vi "QPSK Demodulation (SubVI).vi"(11 "Array in":dynamicdata[](array[waveform])) -> (1 "Output bits":dbl[](array[numeric]), 2 "Constellation graph":cluster{"Y":dbl[], "Y":dbl[]}[](graph), 3 "Even bits":dbl[](graph), 4 "size(s)":i32, 5 "Odd bits":dbl[](graph), 6 "output bits graph":dbl[](graph))   [LabVIEW 2026]
uses:
  <vilib>/measure/madcrms.llb/Basic Averaged DC-RMS for N Chan.vi
  <vilib>/measure/NI_MAPro.lvlib
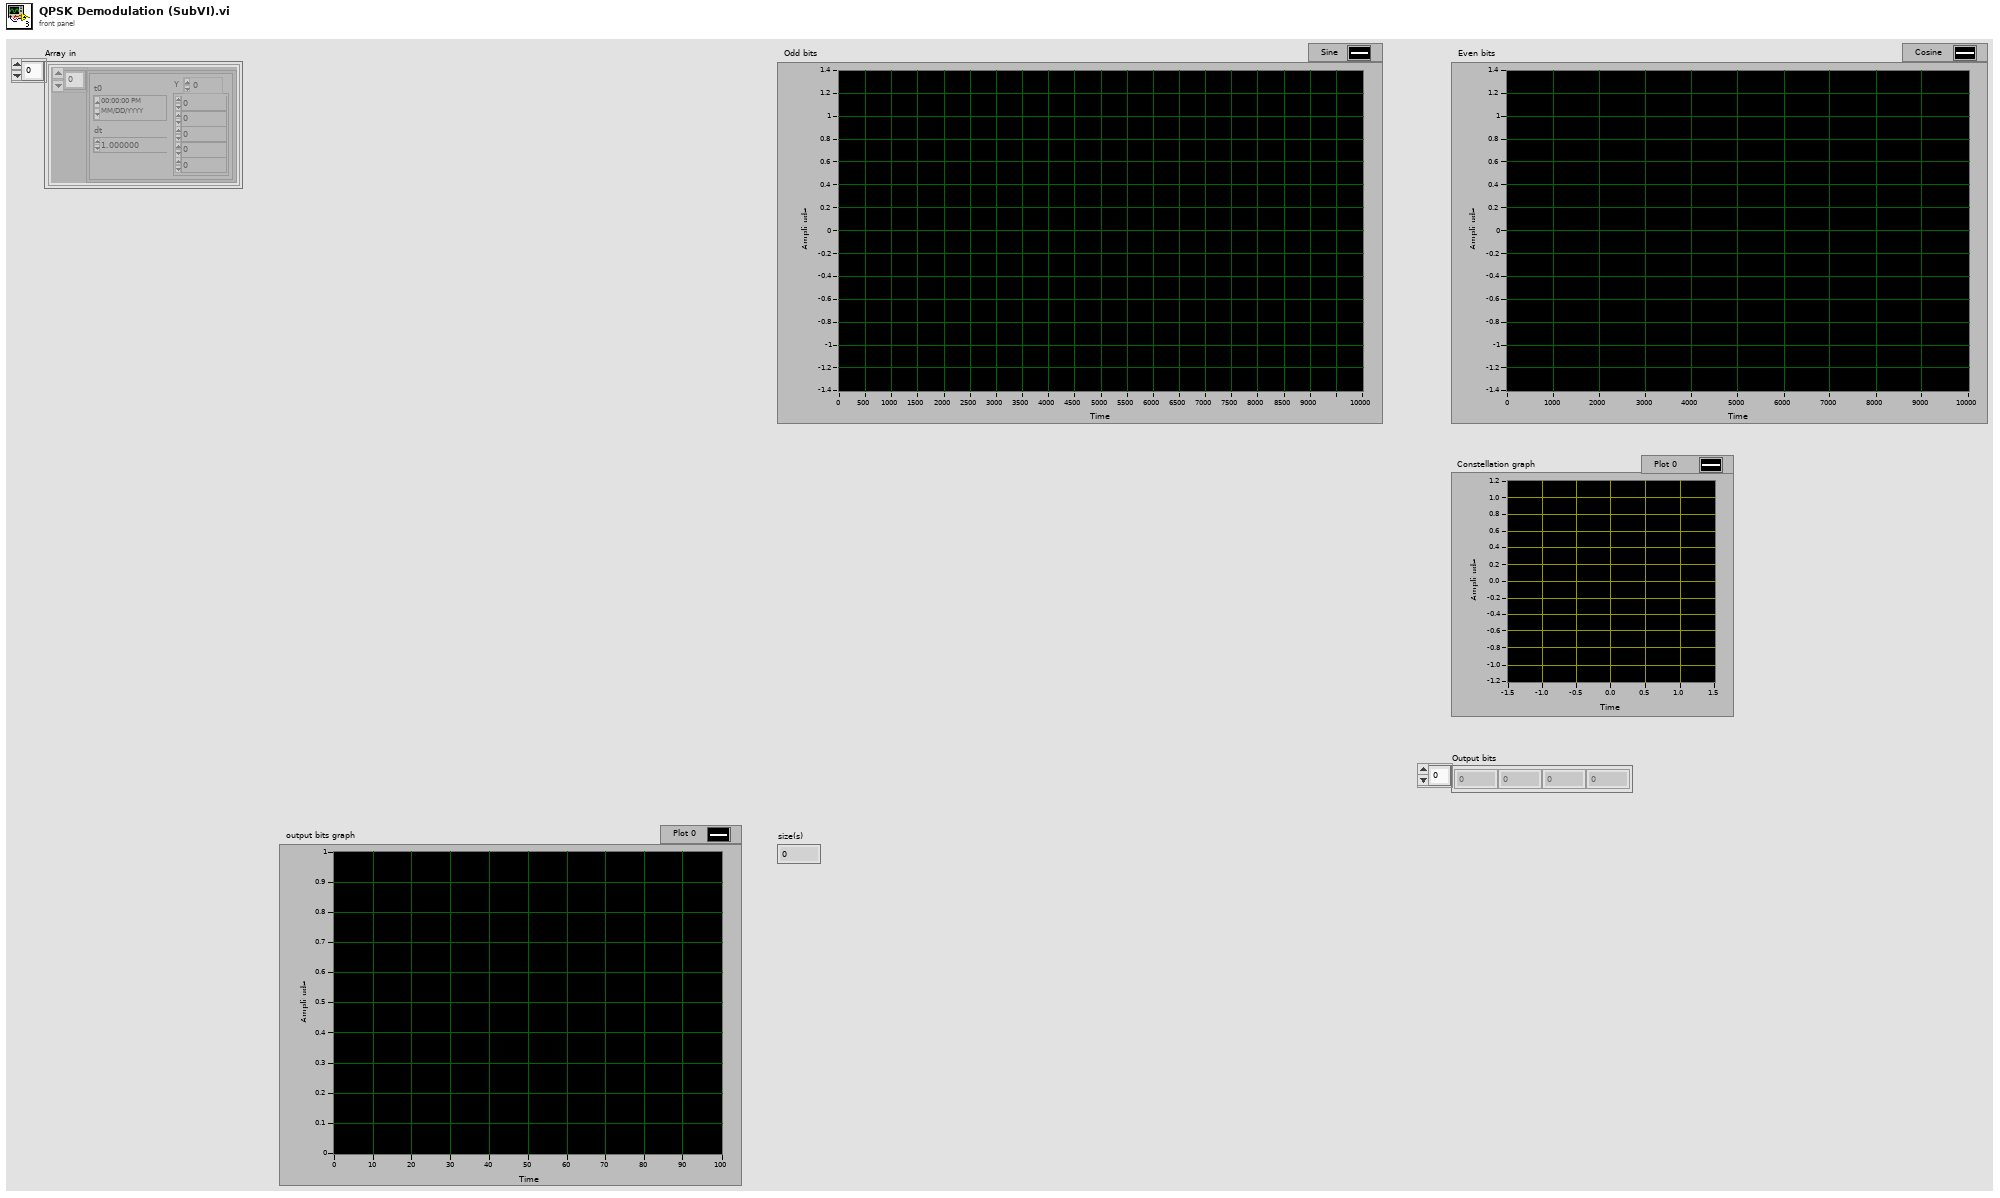
[diagram p1: front panel]
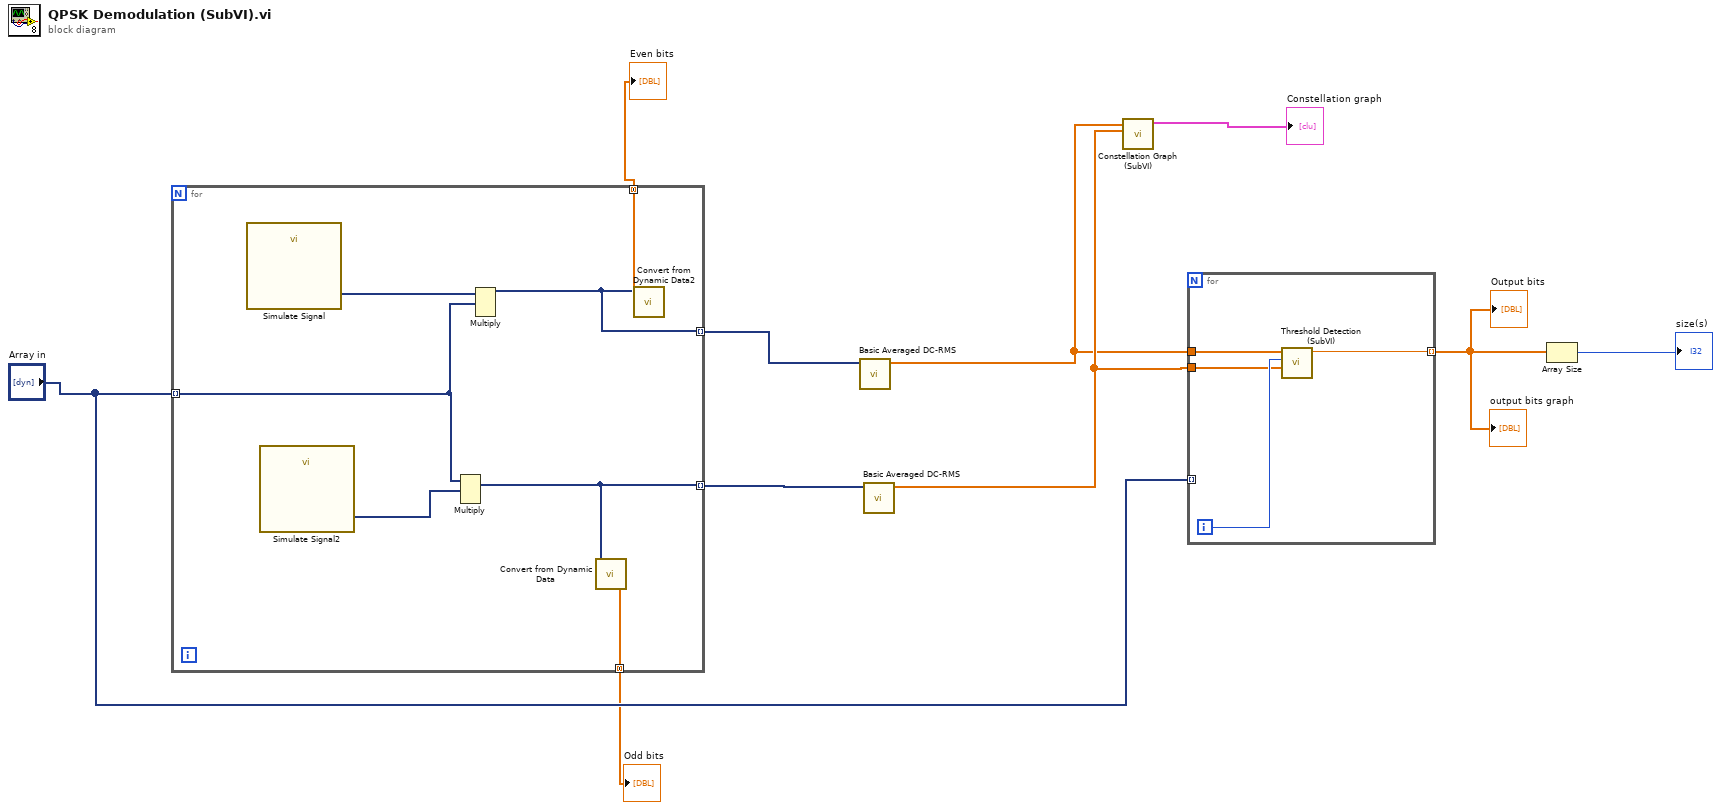
[diagram p0: block diagram]
diagram:
  n1 = for {
    tunnel: "Array in" -> [w15] mode=indexing
    tunnel: [w13] -> w4 mode=concatenating
    tunnel: [w14] -> w3 mode=concatenating
    tunnel: [w12] -> w5 mode=indexing
    tunnel: [w11] -> w6 mode=indexing
    n2 = call "Simulate Signal"() -> ("Cosine"=w17:dynamicdata)  [unwired: 14 in, 1 out]
    n3 = call "Simulate Signal2"() -> ("Sine"=w16:dynamicdata)  [unwired: 14 in, 1 out]
    n4 = Multiply(1:w16, 2:w15) -> (0:w11:dynamicdata)  [unwired: 1 in, 1 out]
    n5 = Multiply(1:w15, 2:w17) -> (0:w12:dynamicdata)  [unwired: 1 in, 1 out]
    n6 = call "Convert from Dynamic Data"("Dynamic Data Type"=w11) -> ("Array"=w14:dbl[])  [unwired: 3 in]
    n7 = call "Convert from Dynamic Data2"("Dynamic Data Type"=w12) -> ("Array"=w13:dbl[])  [unwired: 3 in]
  }
  "Even bits" <- w4
  "Odd bits" <- w3
  n8 = call-poly <vilib>:"Basic Averaged DC-RMS.vi"("signals in"=w5) -> ("DC values"=w7:dbl[])  [unwired: 7 in, 3 out]
  n9 = call-poly <vilib>:"Basic Averaged DC-RMS.vi"("signals in"=w6) -> ("DC values"=w8:dbl[])  [unwired: 7 in, 3 out]
  n10 = call "Constellation Graph (SubVI).vi"("Odd bits"=w8, "Even bits"=w7) -> ("Constellation graph"=→"Constellation graph":cluster{"Y":dbl[], "Y":dbl[]}[])  [unwired: 9 in]
  n11 = for {
    tunnel: w7 -> [w20]
    tunnel: w8 -> [w19]
    tunnel: "Array in" -> [_] mode=indexing
    tunnel: [w18] -> w10 mode=indexing
    i -> [w21]
    n12 = call "Threshold Detection (SubVI).vi"("Array 2"=w19, "index"=w21, "Array"=w20) -> ("Output"=w18:dbl)  [unwired: 8 in]
  }
  "Output bits" <- w10
  "output bits graph" <- w10
  n13 = Array Size(array=w10) -> (size(s)=→"size(s)":i32)
